vi "detected_conversion.vi"(9 "Offset":dbl, 11 "Voltage":string) -> (3 "Optical Power":string)   [LabVIEW 2017]
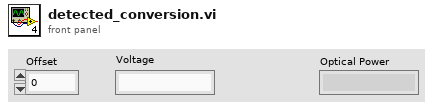
[diagram p1: front panel]
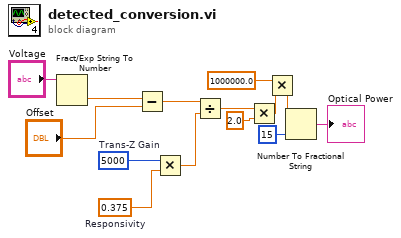
[diagram p0: block diagram]
diagram:
  w12 = 0.375  # Responsivity
  w13 = 5000  # Trans-Z Gain
  n1 = Fract/Exp String To Number(string="Voltage") -> (number=w2:dbl)  [unwired: 3 in, 1 out]
  n2 = Subtract(x=w2, y="Offset") -> (x-y=w3:dbl)
  n3 = Multiply(x=w13, y=w12) -> (x*y=w11:dbl)
  n4 = Divide(x=w3, y=w11) -> (x/y=w9:dbl)
  n5 = Multiply(x=w9, y=2.0) -> (x*y=w5:dbl)
  n6 = Multiply(x=1000000.0, y=w5) -> (x*y=w6:dbl)
  n7 = Number To Fractional String(number=w6, precision (6)=i16 15) -> (F-format string=→"Optical Power":string)  [unwired: 2 in]
